vi "Messaging DeQ.vi"(6 "Time out":i32=100, 8 "Error In":errorcluster) -> (0 "error out":errorcluster, 3 "Data":variant, 4 "Command":string, 5 "[String Data]":string[](array[string]))   [LabVIEW 2019, in "GUI.lvlib"]
doc: "Removes the most recent element from the Queue."
uses:
  GUI.lvlib
  Controls/Messaging Actions.ctl
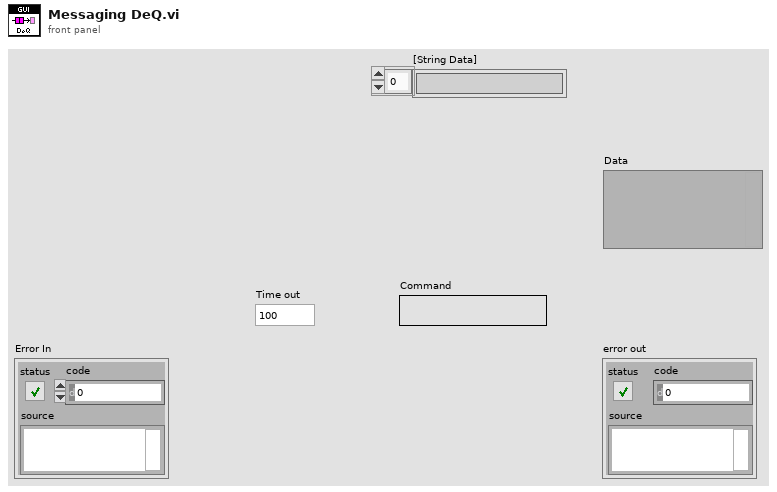
[diagram p1: front panel]
types:
  T1 = typedef "GUI.lvlib/Messaging Actions.ctl" = enum16{"Create", "Get", "Destroy"}
  T2 = typedef "Module Template.lvlib/Message Data.ctl" = cluster{"Command":string, "Data":variant}
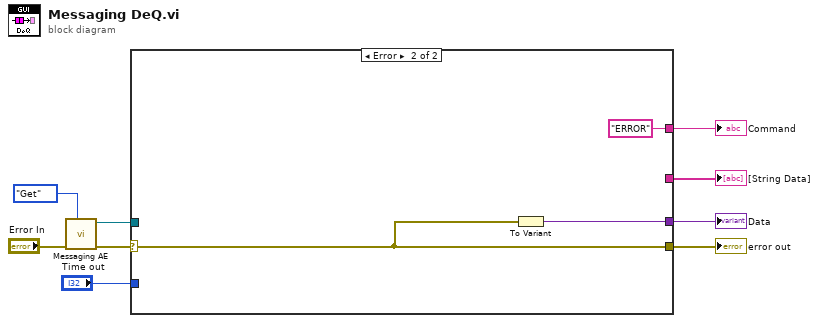
[diagram p0: block diagram]
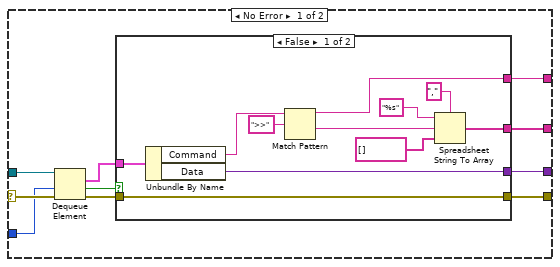
[diagram p2: hidden frame]
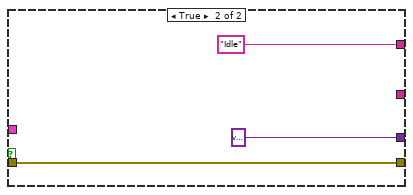
[diagram p3: hidden frame]
diagram:
  n1 = call "Messaging AE.vi"("Action"=Messaging_Actions."Get", "Error In"="Error In") -> ("Error Out"=w4:errorcluster, "queue out"=w3:refnum<queue>)  [unwired: 8 in]
  n2 = case shown="Error" w4 {
    selector: w4 -> [w11 w35]
    tunnel: [w18 "ERROR" ("Command")] -> w1
    tunnel: [w17 w34] -> w8
    tunnel: [w16 w35] -> w7
    tunnel: [w13 _] -> w5
    tunnel: w3 -> [w12 _]
    tunnel: "Time out" -> [w10 _]
    frame No Error {
      n3 = Dequeue Element(queue=w12, timeout in ms (-1)=w10, error in (no error)=w11) -> (element=w19:T2, timed out?=w14:bool, error out=w15:errorcluster)  [unwired: 1 out]
      n4 = case shown="False" w14 {
        tunnel: w19 -> [w30 _]
        tunnel: [w25 "Idle" ("Command")] -> w18
        tunnel: [w29 variant ("Data")] -> w17
        tunnel: [w28 w33] -> w16
        tunnel: w15 -> [w28 w33]
        tunnel: [w21 _] -> w13
        frame False {
          n5 = Unbundle By Name(w30) -> ("Command"=w27:string, "Data"=w29:variant)
          n6 = Match Pattern(string=w27, regular expression=">>") -> (before substring=w25:string, after substring=w24:string)  [unwired: 1 in, 2 out]
          n7 = Spreadsheet String To Array(delimiter (Tab)="," ("format string"), format string="%s", spreadsheet string=w24, array type (2D Dbl)=string[] []) -> (array=w21:string[])
        }
        frame True {
        }
      }
    }
    frame Error {
      n8 = To Variant(anything=w35) -> (Variant=w34:variant)
    }
  }
  "Command" <- w1
  "Data" <- w8
  "error out" <- w7
  "[String Data]" <- w5
